vi "Anritsu VNA Fetch Data.vi"(4 "Trace":i8=1 min=1 max=99 step=1, 5 "Number of Points":i32, 6 "Channel":i8=1 min=1 max=99 step=1, 7 "Anritsu VNA":T1, 8 "error in (no error)":errorcluster, 9 "Formatted Data?":bool, 10 "Data to Read (Data)":enum16{"Data", "Memory"}(ring), 11 "VISA Resource Name":refnum<visa-resource-name>) -> (0 "error out":errorcluster, 2 "Data (real+imag)":cdb[](array[numeric]) format="%#.3f", 3 "dup VISA Resource Name":refnum<visa-resource-name>)   [LabVIEW 2011]
doc: "It is recommended that you hold off triggers before running this VI as the HP8753 tends to \"hang\" if data is read while measurements are being taken.\n\n This VI is used to collect and display data generated by the HP8753 Network Analyzer. The VI can display error-corrected data, error-corrected trace memory, fully formatted data and memory traces. For further information on these types of data see Processsing Chain figure in the HPIB programming note. When the data type is a formatted data, the instruments screen will change to reflect what is being displayed, eg. selecting \"formatted memory\" changes the display to \"MEMORY\".\n\n The data values shown depend upon the data type and the measurement format. If the data type is \"error-corrected data\" or \"error-corrected trace memory\" and/or the measurement format is \"Smith chart\" or \"polar\", the data values are real,imaginary pairs. Otherwise the data values are stimulus,response pairs. These pairs correspond to what is shown in the graphical display.\n\n Data can also be saved to a file with this VI. When saving a file, the stimulus is always shown. The real,imaginary components or the response value are also shown depending upon the data type and the measurement format. \n\n No units are shown on the VI front panel or in the data file. All units are basic units of Hz, dB, seconds, ohms, etc. The \"saved data comments\" control should be used for any special information such as the measurement format, averaging and smoothing information, etc.\n\n Whether or not data is saved and whether the output is in real,imaginary pairs or stimulus,response parirs affects the speed of this VI. When data is saved to a file and/or when data is in stimulus,response pairs, requires the reading of the stimulus values which slows the VI down. The fastest reads are done when the data type is \"error-corrected data\" or \"error-corrected trace memory\" and/or the measurement format is \"Smith chart\" or \"polar\" and data is not being saved to a file.\n\n This VI sets the format, ie. linear or logarithmic, depending upon the sweep type. \n\nFYI - Originally this VI was written without considering the stimulus values. In most case this would be fine for display purposes as the point number could be used for the X value as most sweeps are evenly spaced. This is not the case with frequency list sweeps which can have big gaps in the sweep. For this reason the stimulus value is read (at least in the cases explained above) to make the LabVIEW display match what is display on the instrument's display."
uses:
  TypeDefs/Anritsu VNA Instrument Info.ctl
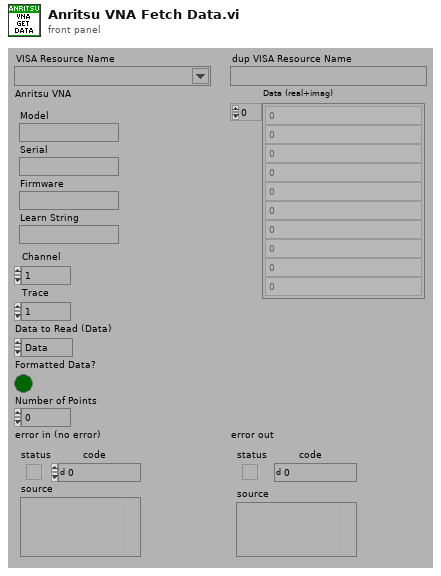
[diagram p1: front panel]
types:
  T1 = typedef "Anritsu VNA Instrument Info.ctl" = cluster{"Model":string, "Serial":string, "Firmware":string, "Learn String":string}
  T2 = typedef "SP Measurement Format.ctl" = enum32{"Log Mag", "Phase", "Delay", "Smith (R+jX)", "Polar (Re/Im)", "Linear Mag", "SWR", "Real", "Imaginary", "Smith (Lin/Phase)", "Smith (Log/Phase)", "Smith (Real/Imag)", "Smith (G+jB)", "Polar (Lin/Phase)", "Polar (Log/Phase)", "Expanded Phase", "Positive Phase", "Inverted Smith", "Unwrapped Phase", "Power Out", "Power In", "Linear Mag/Phase", "Log Mag/Phase", "Real/Imaginary"}
  T3 = typedef "Anritsu VNA Model.ctl" = enum16{"Not Supported", "37XXXX", "MS20XXX", "MS462XX", "MS464XX"}
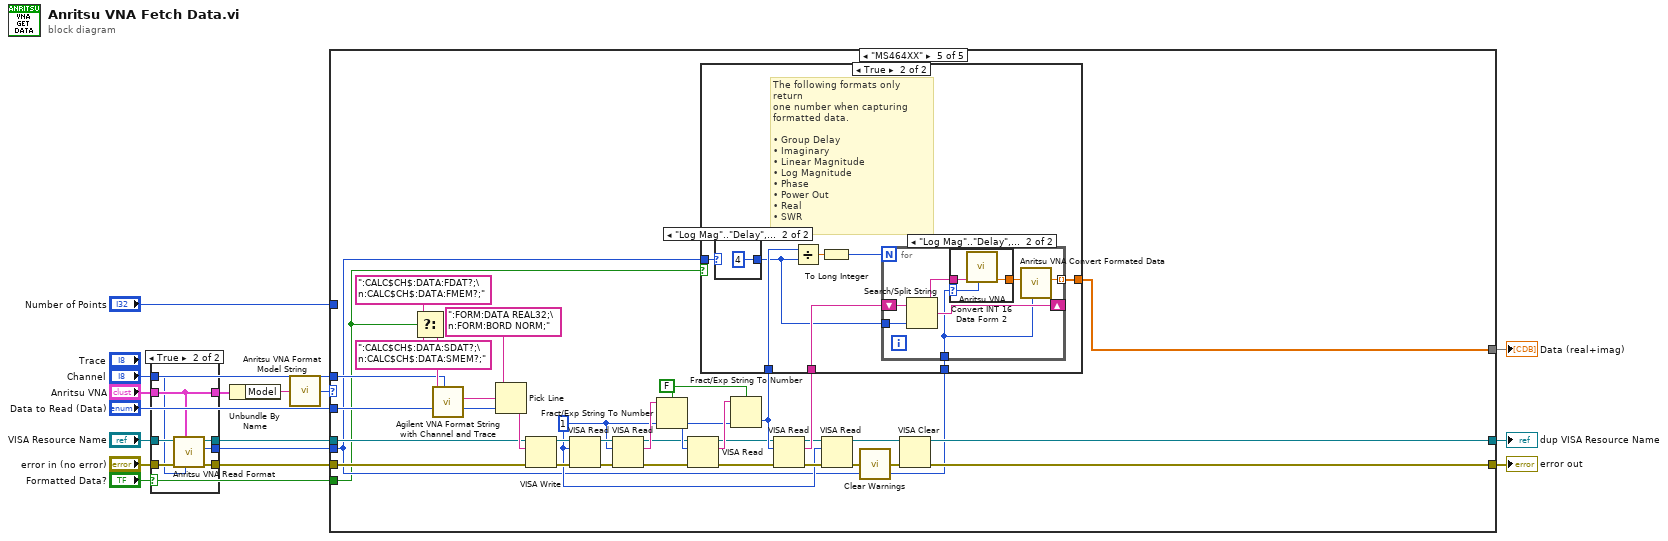
[diagram p0: block diagram]
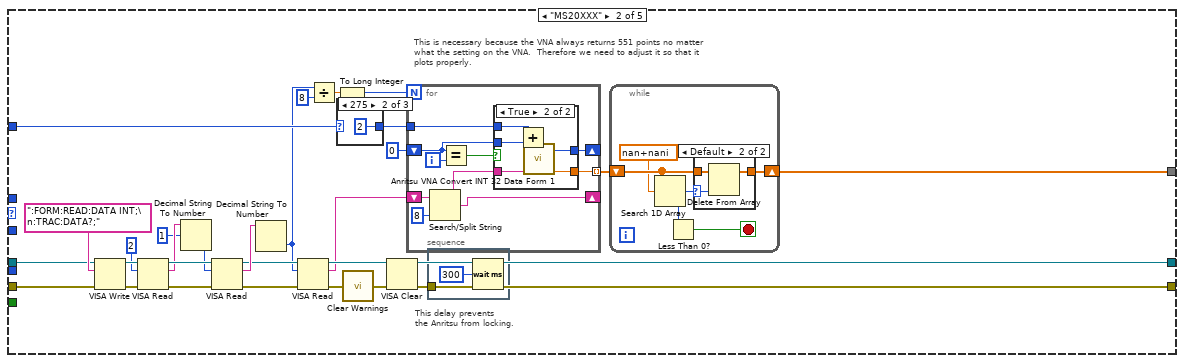
[diagram p4: hidden frame]
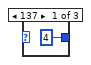
[diagram p6: hidden frame]
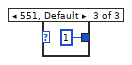
[diagram p7: hidden frame]
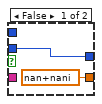
[diagram p8: hidden frame]
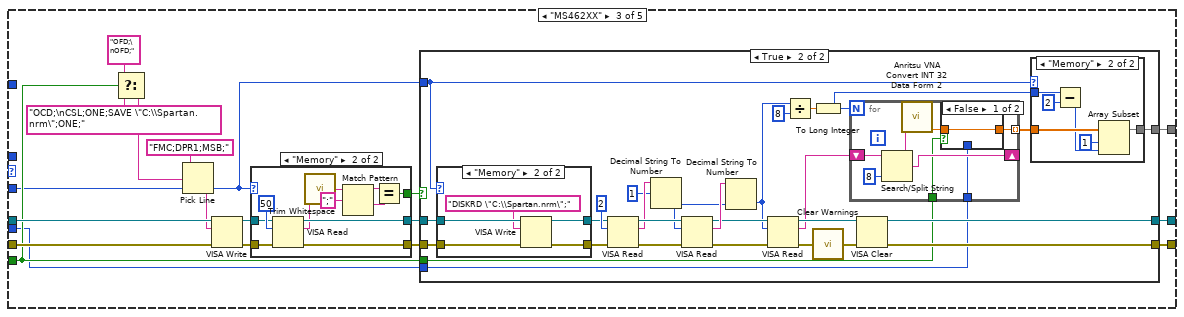
[diagram p9: hidden frame]
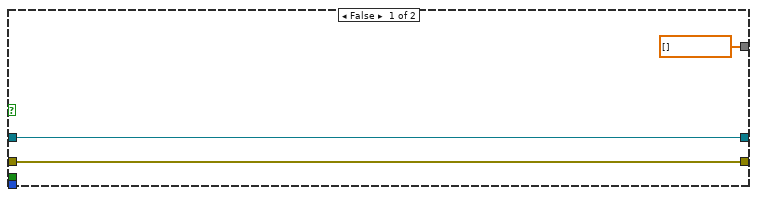
[diagram p10: hidden frame]
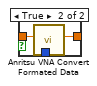
[diagram p13: hidden frame]
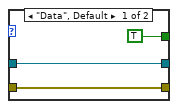
[diagram p14: hidden frame]
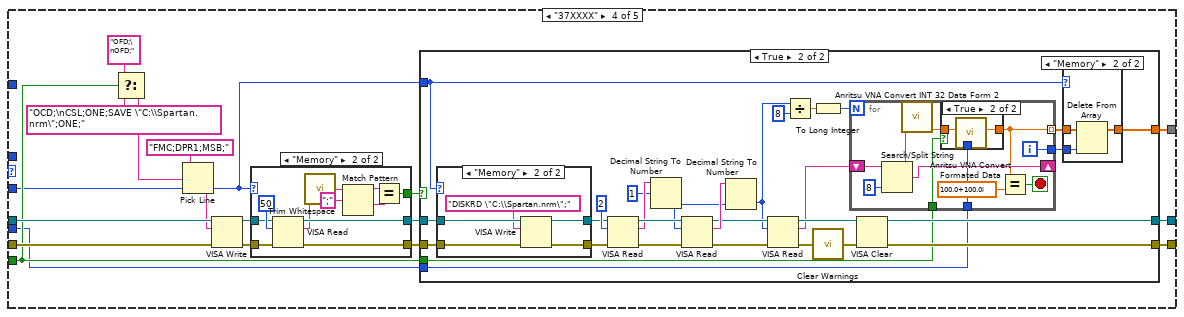
[diagram p15: hidden frame]
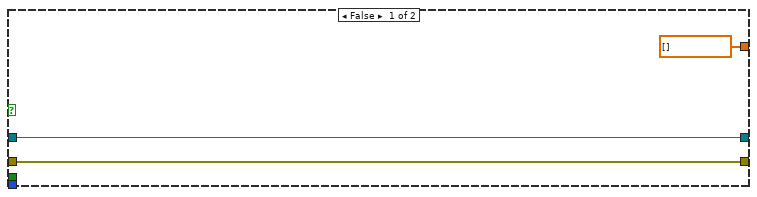
[diagram p16: hidden frame]
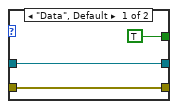
[diagram p20: hidden frame]
diagram:
  n1 = case shown="True" "Formatted Data?" {
    tunnel: "VISA Resource Name" -> [w19 w26]
    tunnel: [w19 w25] -> w11
    tunnel: [w18 w24] -> w10
    tunnel: "error in (no error)" -> [w18 w23]
    tunnel: [_ w22] -> w7
    tunnel: "Anritsu VNA" -> [w17 w21]
    tunnel: [w17 w21] -> w2
    tunnel: "Channel" -> [_ w20]
    frame False {
    }
    frame True {
      n2 = call "Anritsu VNA Read Format.vi"("Channel"=w20, "Anritsu VNA"=w21, "error in (no error)"=w23, "VISA Resource Name"=w26) -> ("error out"=w24:errorcluster, "Display Format"=w22:T2, "dup VISA Resource Name"=w25:refnum<visa-resource-name>)  [unwired: 5 out]
    }
  }
  n3 = Unbundle By Name(w2) -> ("Model"=w5:string)
  n4 = call "Anritsu VNA Format Model String.vi"("Model"=w5) -> ("Model"=w4:T3)
  n5 = case shown="\"MS464XX\"" w4 {
    tunnel: [w28 w29 w102 w191 w289] -> w16
    tunnel: [w27 w52 w105 w194 w288] -> w15
    tunnel: "Formatted Data?" -> [_ _ w95 w184 w267]
    tunnel: [_ w36 w96 w185 w285] -> w6
    tunnel: w10 -> [w28 w42 w104 w193 w291]
    tunnel: w11 -> [w27 w41 w103 w192 w290]
    tunnel: "Number of Points" -> [_ w40 _ _ _]
    tunnel: "Data to Read (Data)" -> [_ _ w93 w182 w287]
    tunnel: w7 -> [_ _ w94 w183 w268]
    tunnel: "Channel" -> [_ _ _ _ w286]
    frame "Not Supported" {
    }
    frame "MS20XXX" {
      # "This delay prevents\nthe Anritsu from locking."
      # "This is necessary because the VNA always returns 551 points no matter\nwhat the setting on the VNA.  Therefore we need to adjust it so that it\nplots properly."
      n6 = VISA Write(VISA resource name=w41, write buffer=":FORM:READ:DATA INT;\n:TRAC:DATA?;" ("String"), error in (no error)=w42) -> (VISA resource name out=w57:refnum<visa-resource-name>, error out=w56:errorcluster)  [unwired: 1 out]
      n7 = VISA Read(VISA resource name=w57, byte count=i8 2, error in (no error)=w56) -> (VISA resource name out=w55:refnum<visa-resource-name>, read buffer=w48:string, error out=w54:errorcluster)  [unwired: 1 out]
      n8 = Decimal String To Number(string=w48, offset=i8 1) -> (number=w46:i32)  [unwired: 2 out]
      n9 = VISA Read(VISA resource name=w55, byte count=w46, error in (no error)=w54) -> (VISA resource name out=w51:refnum<visa-resource-name>, read buffer=w53:string, error out=w50:errorcluster)  [unwired: 1 out]
      n10 = Decimal String To Number(string=w53) -> (number=w32:i32)  [unwired: 1 in, 2 out]
      n11 = VISA Read(VISA resource name=w51, byte count=w32, error in (no error)=w50) -> (VISA resource name out=w49:refnum<visa-resource-name>, read buffer=w44:string, error out=w31:errorcluster)  [unwired: 1 out]
      n12 = Divide(x=w32, y=i8 8) -> (x/y=w34:dbl)
      n13 = To Long Integer(number=w34) -> (32bit integer=w33:i32)
      n14 = case shown="275" w40 {
        tunnel: [i8 4 ("offset (0)") i8 2 ("offset (0)") i8 1 ("offset (0)")] -> w38
        frame 137 {
        }
        frame 275 {
        }
        frame 551, Default {
        }
      }
      n15 = call "Clear Warnings.vi"("error in (no error)"=w31) -> ("error out"=w30:errorcluster)
      n16 = VISA Clear(VISA resource name=w49, error in (no error)=w30) -> (VISA resource name out=w52:refnum<visa-resource-name>, error out=w29:errorcluster)
      n17 = for {
        N: w33 -> [_]
        shift-right: [w78] -> _
        shift-left: w44 -> [w79]
        tunnel: [w76] -> w37 mode=indexing
        shift-right: [w71] -> _
        shift-left: i8 0 ("offset (0)") -> [w72]
        tunnel: w38 -> [w73]
        i -> [w75]
        n18 = Search/Split String(string=w79, offset (0)=i8 8) -> (substring before match=w77:string, match + rest of string=w78:string)  [unwired: 2 out]
        n19 = Equal?(x=w72, y=w75) -> (x = y?=w74:bool)
        n20 = case shown="True" w74 {
          tunnel: w77 -> [_ w87]
          tunnel: [cdb nan+nani ("Number") w86] -> w76
          tunnel: w73 -> [_ w84]
          tunnel: w72 -> [w82 w85]
          tunnel: [w82 w83] -> w71
          frame False {
          }
          frame True {
            n21 = Add(x=w84, y=w85) -> (x+y=w83:i8)
            n22 = call "Anritsu VNA Convert INT 32 Data Form 1.vi"("Raw Data Point"=w87) -> ("Number"=w86:cdb)  [unwired: 10 out]
          }
        }
      }
      n23 = stacked-sequence {
        tunnel: w29 -> [_]
        frame #0 {
          n24 = Wait (ms)(milliseconds to wait=u32 300) -> ()  [unwired: 1 out]
        }
      }
      n25 = while {
        shift-right: [w63] -> w36
        shift-left: w37 -> [w62]
        stop <- w59 stop-if-true
        n26 = Search 1D Array(1D array=w62, element=cdb nan+nani ("Number")) -> (index of element=w60:i32)  [unwired: 1 out]
        n27 = Less Than 0?(x=w60) -> (x < 0?=w59:bool)
        n28 = case shown="Default" w60 {
          selector: w60 -> [_ w65]
          tunnel: w62 -> [w64 w67]
          tunnel: [w64 w66] -> w63
          frame -1 {
          }
          frame Default {
            n29 = Delete From Array(array=w67, index=w65) -> (array with subset deleted=w66:cdb[])  [unwired: 1 in, 1 out]
          }
        }
      }
    }
    frame "MS462XX" {
      n30 = Select(t="OFD;\nOFD;" ("String"), s=w95, f="OCD;\nCSL;ONE;SAVE \"C:\\Spartan.nrm\";ONE;" ("String")) -> (s? t:f=w98:string)
      n31 = Pick Line(string ("")="FMC;DPR1;MSB;" ("String"), multi-line string=w98, line index=w93) -> (output string=w97:string)
      n32 = VISA Write(VISA resource name=w103, write buffer=w97, error in (no error)=w104) -> (VISA resource name out=w92:refnum<visa-resource-name>, error out=w90:errorcluster)  [unwired: 1 out]
      n33 = case shown="\"Memory\"" w93 {
        tunnel: [w165 w175] -> w91
        tunnel: w92 -> [w165 w172]
        tunnel: [w164 w174] -> w89
        tunnel: w90 -> [w164 w173]
        tunnel: [TRUE w166] -> w88
        frame "Data", Default {
        }
        frame "Memory" {
          n34 = VISA Read(VISA resource name=w172, byte count=u32 50, error in (no error)=w173) -> (VISA resource name out=w175:refnum<visa-resource-name>, read buffer=w170:string, error out=w174:errorcluster)  [unwired: 1 out]
          n35 = call <vilib>:"Trim Whitespace.vi"("string"=w170) -> ("trimmed string"=w169:string)  [unwired: 1 in]
          n36 = Match Pattern(string=w169, regular expression=";") -> (before substring=w168:string, after substring=w167:string)  [unwired: 3 out]
          n37 = Equal?(x=w168, y=w167) -> (x = y?=w166:bool)
        }
      }
      n38 = case shown="True" w88 {
        tunnel: [w107 w133] -> w105
        tunnel: [w108 w120] -> w102
        tunnel: [cdb[] [] w118] -> w96
        tunnel: w95 -> [_ w115]
        tunnel: w94 -> [_ w114]
        tunnel: w93 -> [_ w113]
        tunnel: w91 -> [w107 w112]
        tunnel: w89 -> [w108 w111]
        frame False {
        }
        frame True {
          w116 = u32 1
          n39 = case shown="\"Memory\"" w113 {
            tunnel: [w138 w141] -> w110
            tunnel: w112 -> [w138 w142]
            tunnel: [w137 w140] -> w109
            tunnel: w111 -> [w137 w143]
            frame "Data", Default {
            }
            frame "Memory" {
              n40 = VISA Write(VISA resource name=w142, write buffer="DISKRD \"C:\\Spartan.nrm\";" ("regular expression"), error in (no error)=w143) -> (VISA resource name out=w141:refnum<visa-resource-name>, error out=w140:errorcluster)  [unwired: 1 out]
            }
          }
          n41 = VISA Read(VISA resource name=w110, byte count=u32 2, error in (no error)=w109) -> (VISA resource name out=w136:refnum<visa-resource-name>, read buffer=w129:string, error out=w135:errorcluster)  [unwired: 1 out]
          n42 = Decimal String To Number(string=w129, offset=w116, default (0L)=w116) -> (number=w127:u32)  [unwired: 1 out]
          n43 = VISA Read(VISA resource name=w136, byte count=w127, error in (no error)=w135) -> (VISA resource name out=w132:refnum<visa-resource-name>, read buffer=w134:string, error out=w131:errorcluster)  [unwired: 1 out]
          n44 = Decimal String To Number(string=w134, default (0L)=w116) -> (number=w123:u32)  [unwired: 1 in, 1 out]
          n45 = VISA Read(VISA resource name=w132, byte count=w123, error in (no error)=w131) -> (VISA resource name out=w130:refnum<visa-resource-name>, read buffer=w126:string, error out=w122:errorcluster)  [unwired: 1 out]
          n46 = Divide(x=w123, y=8) -> (x/y=w124:dbl)
          n47 = To Long Integer(number=w124) -> (32bit integer=w117:i32)
          n48 = call "Clear Warnings.vi"("error in (no error)"=w122) -> ("error out"=w121:errorcluster)
          n49 = for {
            N: w117 -> [_]
            shift-right: [w156] -> _
            shift-left: w126 -> [w158]
            tunnel: [w153] -> w119 mode=indexing
            tunnel: w115 -> [w152]
            tunnel: w114 -> [w151]
            n50 = Search/Split String(string=w158, offset (0)=i8 8) -> (substring before match=w155:string, match + rest of string=w156:string)  [unwired: 2 out]
            n51 = call "Anritsu VNA Convert INT 32 Data Form 2.vi"("Raw Data Point"=w155) -> ("Number"=w154:cdb)  [unwired: 10 out]
            n52 = case shown="False" w152 {
              tunnel: w154 -> [w159 w162]
              tunnel: [w159 w161] -> w153
              tunnel: w151 -> [_ w160]
              frame False {
              }
              frame True {
                n53 = call "Anritsu VNA Convert Formated Data.vi"("Display Format"=w160, "Number"=w162) -> ("Number"=w161:cdb)  [unwired: 9 out]
              }
            }
          }
          n54 = VISA Clear(VISA resource name=w130, error in (no error)=w121) -> (VISA resource name out=w133:refnum<visa-resource-name>, error out=w120:errorcluster)
          n55 = case shown="\"Memory\"" w113 {
            tunnel: w119 -> [w144 w150]
            tunnel: [w144 w149] -> w118
            tunnel: w117 -> [_ w147]
            frame "Data", Default {
            }
            frame "Memory" {
              n56 = Subtract(x=w147, y=2) -> (x-y=w145:i32)
              n57 = Array Subset(array=w150, index=1, length=w145) -> (w149:cdb[])
            }
          }
        }
      }
    }
    frame "37XXXX" {
      n58 = Select(t="OFD;\nOFD;" ("String"), s=w184, f="OCD;\nCSL;ONE;SAVE \"C:\\Spartan.nrm\";ONE;" ("String")) -> (s? t:f=w187:string)
      n59 = Pick Line(string ("")="FMC;DPR1;MSB;" ("String"), multi-line string=w187, line index=w182) -> (output string=w186:string)
      n60 = VISA Write(VISA resource name=w192, write buffer=w186, error in (no error)=w193) -> (VISA resource name out=w181:refnum<visa-resource-name>, error out=w179:errorcluster)  [unwired: 1 out]
      n61 = case shown="\"Memory\"" w182 {
        tunnel: [w255 w265] -> w180
        tunnel: w181 -> [w255 w262]
        tunnel: [w254 w264] -> w178
        tunnel: w179 -> [w254 w263]
        tunnel: [TRUE w256] -> w177
        frame "Data", Default {
        }
        frame "Memory" {
          n62 = VISA Read(VISA resource name=w262, byte count=u32 50, error in (no error)=w263) -> (VISA resource name out=w265:refnum<visa-resource-name>, read buffer=w260:string, error out=w264:errorcluster)  [unwired: 1 out]
          n63 = call <vilib>:"Trim Whitespace.vi"("string"=w260) -> ("trimmed string"=w259:string)  [unwired: 1 in]
          n64 = Match Pattern(string=w259, regular expression=";") -> (before substring=w258:string, after substring=w257:string)  [unwired: 3 out]
          n65 = Equal?(x=w258, y=w257) -> (x = y?=w256:bool)
        }
      }
      n66 = case shown="True" w177 {
        tunnel: [w196 w223] -> w194
        tunnel: [w197 w210] -> w191
        tunnel: [cdb[] [] w208] -> w185
        tunnel: w184 -> [_ w206]
        tunnel: w183 -> [_ w205]
        tunnel: w182 -> [_ w204]
        tunnel: w180 -> [w196 w203]
        tunnel: w178 -> [w197 w202]
        frame False {
        }
        frame True {
          w207 = u32 1
          n67 = case shown="\"Memory\"" w204 {
            tunnel: [w228 w231] -> w201
            tunnel: w203 -> [w228 w232]
            tunnel: [w227 w230] -> w200
            tunnel: w202 -> [w227 w233]
            frame "Data", Default {
            }
            frame "Memory" {
              n68 = VISA Write(VISA resource name=w232, write buffer="DISKRD \"C:\\Spartan.nrm\";" ("regular expression"), error in (no error)=w233) -> (VISA resource name out=w231:refnum<visa-resource-name>, error out=w230:errorcluster)  [unwired: 1 out]
            }
          }
          n69 = VISA Read(VISA resource name=w201, byte count=u32 2, error in (no error)=w200) -> (VISA resource name out=w226:refnum<visa-resource-name>, read buffer=w219:string, error out=w225:errorcluster)  [unwired: 1 out]
          n70 = Decimal String To Number(string=w219, offset=w207, default (0L)=w207) -> (number=w217:u32)  [unwired: 1 out]
          n71 = VISA Read(VISA resource name=w226, byte count=w217, error in (no error)=w225) -> (VISA resource name out=w222:refnum<visa-resource-name>, read buffer=w224:string, error out=w221:errorcluster)  [unwired: 1 out]
          n72 = Decimal String To Number(string=w224, default (0L)=w207) -> (number=w213:u32)  [unwired: 1 in, 1 out]
          n73 = VISA Read(VISA resource name=w222, byte count=w213, error in (no error)=w221) -> (VISA resource name out=w220:refnum<visa-resource-name>, read buffer=w216:string, error out=w212:errorcluster)  [unwired: 1 out]
          n74 = Divide(x=w213, y=8) -> (x/y=w214:dbl)
          n75 = To Long Integer(number=w214) -> (32bit integer=w199:i32)
          n76 = call "Clear Warnings.vi"("error in (no error)"=w212) -> ("error out"=w211:errorcluster)
          n77 = for {
            N: w199 -> [_]
            shift-right: [w246] -> _
            shift-left: w216 -> [w248]
            tunnel: [w241] -> w209 mode=indexing
            tunnel: w206 -> [w243]
            tunnel: w205 -> [w242]
            tunnel: [w238] -> w198
            i -> [w238]
            stop <- w239 stop-if-true
            n78 = Search/Split String(string=w248, offset (0)=i8 8) -> (substring before match=w245:string, match + rest of string=w246:string)  [unwired: 2 out]
            n79 = call "Anritsu VNA Convert INT 32 Data Form 2.vi"("Raw Data Point"=w245) -> ("Number"=w244:cdb)  [unwired: 10 out]
            n80 = case shown="True" w243 {
              tunnel: w244 -> [w249 w252]
              tunnel: [w249 w251] -> w241
              tunnel: w242 -> [_ w250]
              frame False {
              }
              frame True {
                n81 = call "Anritsu VNA Convert Formated Data.vi"("Display Format"=w250, "Number"=w252) -> ("Number"=w251:cdb)  [unwired: 9 out]
              }
            }
            n82 = Equal?(x=w241, y=cdb 100.0+100.0i ("Number")) -> (x = y?=w239:bool)
          }
          n83 = VISA Clear(VISA resource name=w220, error in (no error)=w211) -> (VISA resource name out=w223:refnum<visa-resource-name>, error out=w210:errorcluster)
          n84 = case shown="\"Memory\"" w204 {
            tunnel: w209 -> [w234 w237]
            tunnel: [w234 w236] -> w208
            tunnel: w198 -> [_ w235]
            frame "Data", Default {
            }
            frame "Memory" {
              n85 = Delete From Array(array=w237, index=w235) -> (array with subset deleted=w236:cdb[])  [unwired: 1 in, 1 out]
            }
          }
        }
      }
    }
    frame "MS464XX" {
      w269 = u32 1
      w283 = FALSE ("use system decimal point (T)")
      n86 = Select(t=":CALC$CH$:DATA:FDAT?;\n:CALC$CH$:DATA:FMEM?;" ("String"), s=w267, f=":CALC$CH$:DATA:SDAT?;\n:CALC$CH$:DATA:SMEM?;" ("String")) -> (s? t:f=w300:string)
      n87 = call "Agilent VNA Format String with Channel and Trace.vi"("Channel"=w286, "String"=w300) -> ("String Out"=w292:string)  [unwired: 1 in, 6 out]
      n88 = Pick Line(string ("")=":FORM:DATA REAL32;\n:FORM:BORD NORM;" ("String"), multi-line string=w292, line index=w287) -> (output string=w294:string)
      n89 = VISA Write(VISA resource name=w290, write buffer=w294, error in (no error)=w291) -> (VISA resource name out=w278:refnum<visa-resource-name>, error out=w279:errorcluster)  [unwired: 1 out]
      n90 = VISA Read(VISA resource name=w278, byte count=w269, error in (no error)=w279) -> (VISA resource name out=w281:refnum<visa-resource-name>, error out=w280:errorcluster)  [unwired: 2 out]
      n91 = VISA Read(VISA resource name=w281, byte count=w269, error in (no error)=w280) -> (VISA resource name out=w277:refnum<visa-resource-name>, read buffer=w284:string, error out=w276:errorcluster)  [unwired: 1 out]
      n92 = Fract/Exp String To Number(use system decimal point (T)=w283, string=w284, default (0 dbl)=w269) -> (number=w282:u32)  [unwired: 2 out]
      n93 = VISA Read(VISA resource name=w277, byte count=w282, error in (no error)=w276) -> (VISA resource name out=w270:refnum<visa-resource-name>, read buffer=w295:string, error out=w271:errorcluster)  [unwired: 1 out]
      n94 = Fract/Exp String To Number(use system decimal point (T)=w283, string=w295, default (0 dbl)=w269) -> (number=w296:u32)  [unwired: 2 out]
      n95 = VISA Read(VISA resource name=w270, byte count=w296, error in (no error)=w271) -> (VISA resource name out=w273:refnum<visa-resource-name>, read buffer=w297:string, error out=w272:errorcluster)  [unwired: 1 out]
      n96 = case shown="True" w267 {
        tunnel: w297 -> [w307 w320]
        tunnel: w296 -> [w306 w319]
        tunnel: [w303 w316] -> w285
        tunnel: w268 -> [_ w314]
        tunnel: w268 -> [_ w313]
        frame False {
          w302 = 8
          n97 = Divide(x=w306, y=w302) -> (x/y=w304:dbl)
          n98 = To Long Integer(number=w304) -> (32bit integer=w305:i32)
          n99 = for {
            N: w305 -> [_]
            shift-right: [w311] -> _
            shift-left: w307 -> [w312]
            tunnel: [w308] -> w303 mode=indexing
            tunnel: w302 -> [w309]
            n100 = Search/Split String(string=w312, offset (0)=w309) -> (substring before match=w310:string, match + rest of string=w311:string)  [unwired: 2 out]
            n101 = call "Anritsu VNA Convert INT 32 Data Form 2.vi"("Raw Data Point"=w310) -> ("Number"=w308:cdb)  [unwired: 10 out]
          }
        }
        frame True {
          # "The following formats only return\none number when capturing\nformatted data.\n\n• Group Delay\n• Imaginary\n• Linear Magnitude\n• Log Magnitude\n• Phase\n• Power Out\n• Real\n• SWR"
          n102 = case shown="\"Log Mag\"..\"Delay\", \"Linear Mag\"..\"Imaginary\", \"Power Out\"" w314 {
            tunnel: [8 4] -> w315
            frame Default {
            }
            frame "Log Mag".."Delay", "Linear Mag".."Imaginary", "Power Out" {
            }
          }
          n103 = Divide(x=w319, y=w315) -> (x/y=w317:dbl)
          n104 = To Long Integer(number=w317) -> (32bit integer=w318:i32)
          n105 = for {
            N: w318 -> [_]
            shift-right: [w328] -> _
            shift-left: w320 -> [w329]
            tunnel: [w327] -> w316 mode=indexing
            tunnel: w315 -> [w326]
            tunnel: w313 -> [w323]
            n106 = Search/Split String(string=w329, offset (0)=w326) -> (substring before match=w324:string, match + rest of string=w328:string)  [unwired: 2 out]
            n107 = case shown="\"Log Mag\"..\"Delay\", \"Linear Mag\"..\"Imaginary\", \"Power Out\"" w323 {
              selector: w323 -> [_ w333]
              tunnel: [w331 w334] -> w325
              tunnel: w324 -> [w330 w332]
              frame Default {
                n108 = call "Anritsu VNA Convert INT 32 Data Form 2.vi"("Raw Data Point"=w330) -> ("Number"=w331:cdb)  [unwired: 10 out]
              }
              frame "Log Mag".."Delay", "Linear Mag".."Imaginary", "Power Out" {
                n109 = call "Anritsu VNA Convert INT 16 Data Form 2.vi"("Display Format"=w333, "Raw Data Point"=w332) -> ("Number"=w334:cdb)  [unwired: 9 out]
              }
            }
            n110 = call "Anritsu VNA Convert Formated Data.vi"("Display Format"=w323, "Number"=w325) -> ("Number"=w327:cdb)  [unwired: 9 out]
          }
        }
      }
      n111 = VISA Read(VISA resource name=w273, byte count=w269, error in (no error)=w272) -> (VISA resource name out=w274:refnum<visa-resource-name>, error out=w275:errorcluster)  [unwired: 2 out]
      n112 = call "Clear Warnings.vi"("error in (no error)"=w275) -> ("error out"=w301:errorcluster)
      n113 = VISA Clear(VISA resource name=w274, error in (no error)=w301) -> (VISA resource name out=w288:refnum<visa-resource-name>, error out=w289:errorcluster)
    }
  }
  "dup VISA Resource Name" <- w15
  "error out" <- w16
  "Data (real+imag)" <- w6
